vi "PID control.vi"() -> ()   [LabVIEW 2023]
doc: "DESCRIPTION:\n\nThis VI configures the power supply to generate a DC voltage output.\nIt also displays the Output Voltage,Current and Power as per the selected parameter. \n\nINSTRUCTIONS:\n1. Enter the resource name.\n2. Select the desired Channel.\n3. Enter voltage or current value to set the voltage or current value of the power supply .\n4. Set On/Off switch to Enable if you want the generated voltage to appear at the instrument's output. \n5. Select Local/Remote mode operation.If local command is select ,this will set the instrument in local mode.\n6.Select the parameter from the control,to read the responce from the instrument.\n7.Run the VI.\n\nNOTES:\nNotice the order of the power supply component VIs in the block diagram. The first VI in a sequence is the power supply Initialize.vi, which provides a VISA session to the instrument driver. The last VI in a sequence must be the power supply Close.vi which closes the Visa session."
uses:
  <vilib>/Utility/error.llb/DialogType.ctl
  <vilib>/DAQmx/write.llb/DAQmx Write (Digital Bool 1Line 1Point).vi
  <vilib>/DAQmx/read.llb/DAQmx Read (Analog DBL 1Chan 1Samp).vi
  <vilib>/DAQmx/create/channels.llb/DAQmx Create Channel (DO-Digital Output).vi
  <vilib>/DAQmx/miscellaneous.llb/DAQmx Fill In Error Info.vi
  <vilib>/DAQmx/create/channels.llb/DAQmx Create Channel (AI-Voltage-Basic).vi
  <vilib>/addons/control/pid/pid.llb/PID Advanced (DBL).vi
  Downloads/KeithleyKE22xxSeriesVer1.2 (1)/Keithley KE22xx Series/Keithley KE22xx Series.lvlib
  <vilib>/addons/control/pid/NI_PID_pid.lvlib
panel:
  out "message":string=" INSTRUCTIONS:\r\rNormal Use:  When using subVIs that incorporate the error in/error out (or error I/O) structure, place this handler where you want to inform the user of an error, typically at the end of the I/O data path, as the last action of the program.  If the error in error? is ERROR, the handler creates a message describing the error and its source.  If the type of dialog = 1 (default), the message is displayed to the user, who can only acknowedge it.  If the type = 2, the user can acknowledge the message or abort execution; aborting a program with active I/O is not recommended.  If the type = 0, no message is displayed; this is used to process the error programmatically, and the error out cluster elements are wired to individual terminals for that reason.  \r\rOther Use:\n\r\nlocal testing.  To test the error code of a subVI or function that does not have the error I/O structure, you can wire its error code and a source string to the local error code and error source inputs.  If error in error? indicates no error and error code is not equal to 0, the local code and source are substituted for the error in values, and error? is set TRUE (ERROR)."
  in  "stop 2":bool
  out "Temperature [Celsius]\n]":dbl
  in  "Set point Temp [Celsius].":dbl(slide) scale=0.0..40.0
  in  "PID gains in":T1={"proportional gain (Kc)"=1.0, "integral time (Ti, min)"=0.01, "derivative time (Td, min)"=0.0} {"derivative time (Td, min)" format="%.3f"; "integral time (Ti, min)" format="%.3f"; "proportional gain (Kc)" format="%.3f"}
  out "Waveform Chart":T2(graph)
  in  "Channel Select":enum16{"Channel 1", "Channel 2", "Channel 3"}(ring)
  in  "Measurement Function(0:Voltage)":u16(ring) items=["Voltage", "Current", "Power"]
  in  "Function(0:Voltage)":u16(ring) items=["Voltage", "Current"]
  in  "Control Mode(1:Remote)":u16(ring)=1 items=["Local", "Remote"]
  in  "Enable Output (T: Enable)":bool=TRUE
  in  "Unit(V)":u16(ring) items=["V", "mV", "kV", "A", "mA"]
  out "Measurement":string
  in  "VISA resource name":refnum<visa-resource-name>
  # "© 2012 Keithley Instruments, Inc. ALL RIGHTS RESERVED"
  # "Configure Instrument"
  # "Read Measurement"
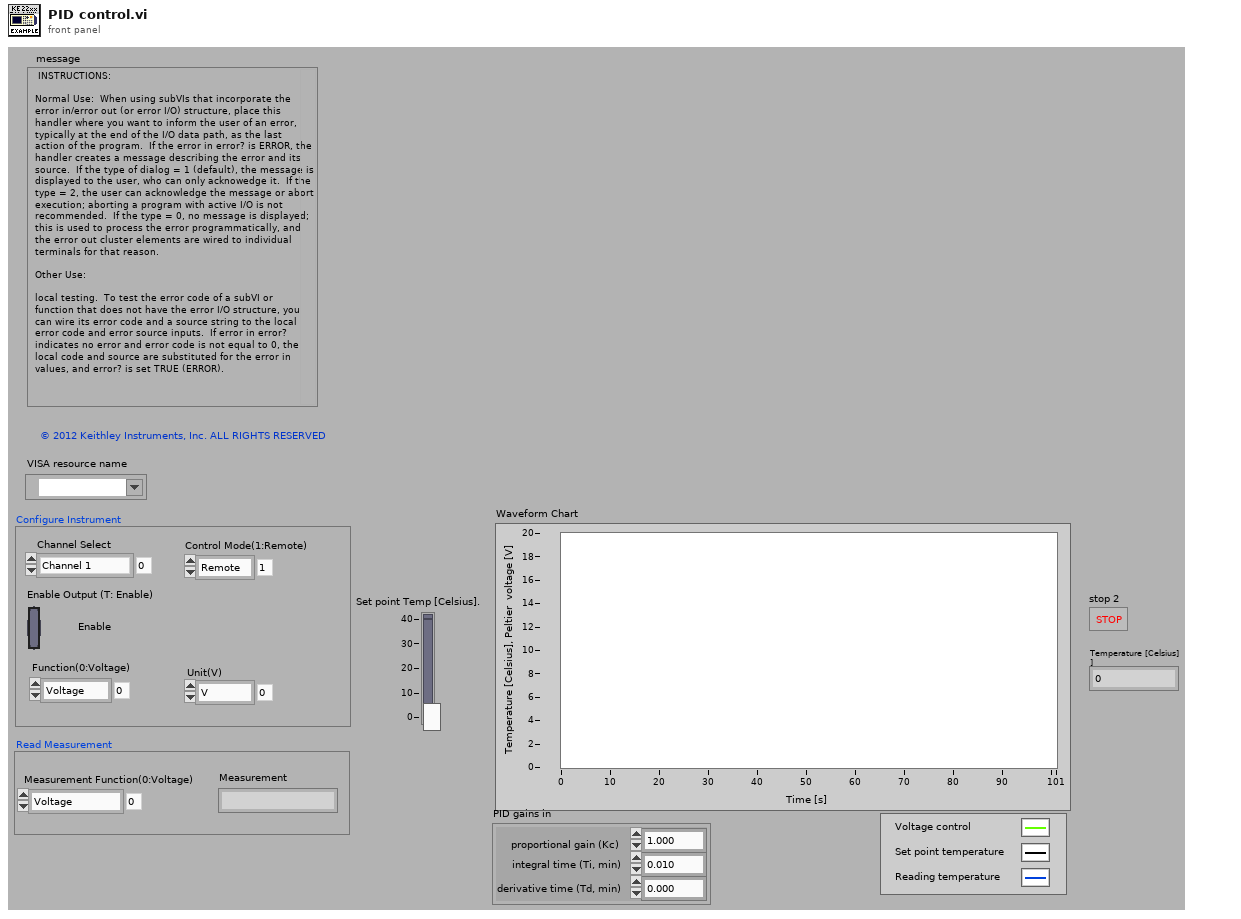
[diagram p1: front panel]
types:
  T1 = cluster{"proportional gain (Kc)":dbl, "integral time (Ti, min)":dbl, "derivative time (Td, min)":dbl}
  T2 = cluster{"Fan Speed":dbl, "Set point Temperature":dbl, "Plant Output":dbl}
  T3 = typedef "DialogType.ctl" = u16
  T4 = cluster{"output":dbl, "Set point Temp [Celsius].":dbl, dbl}
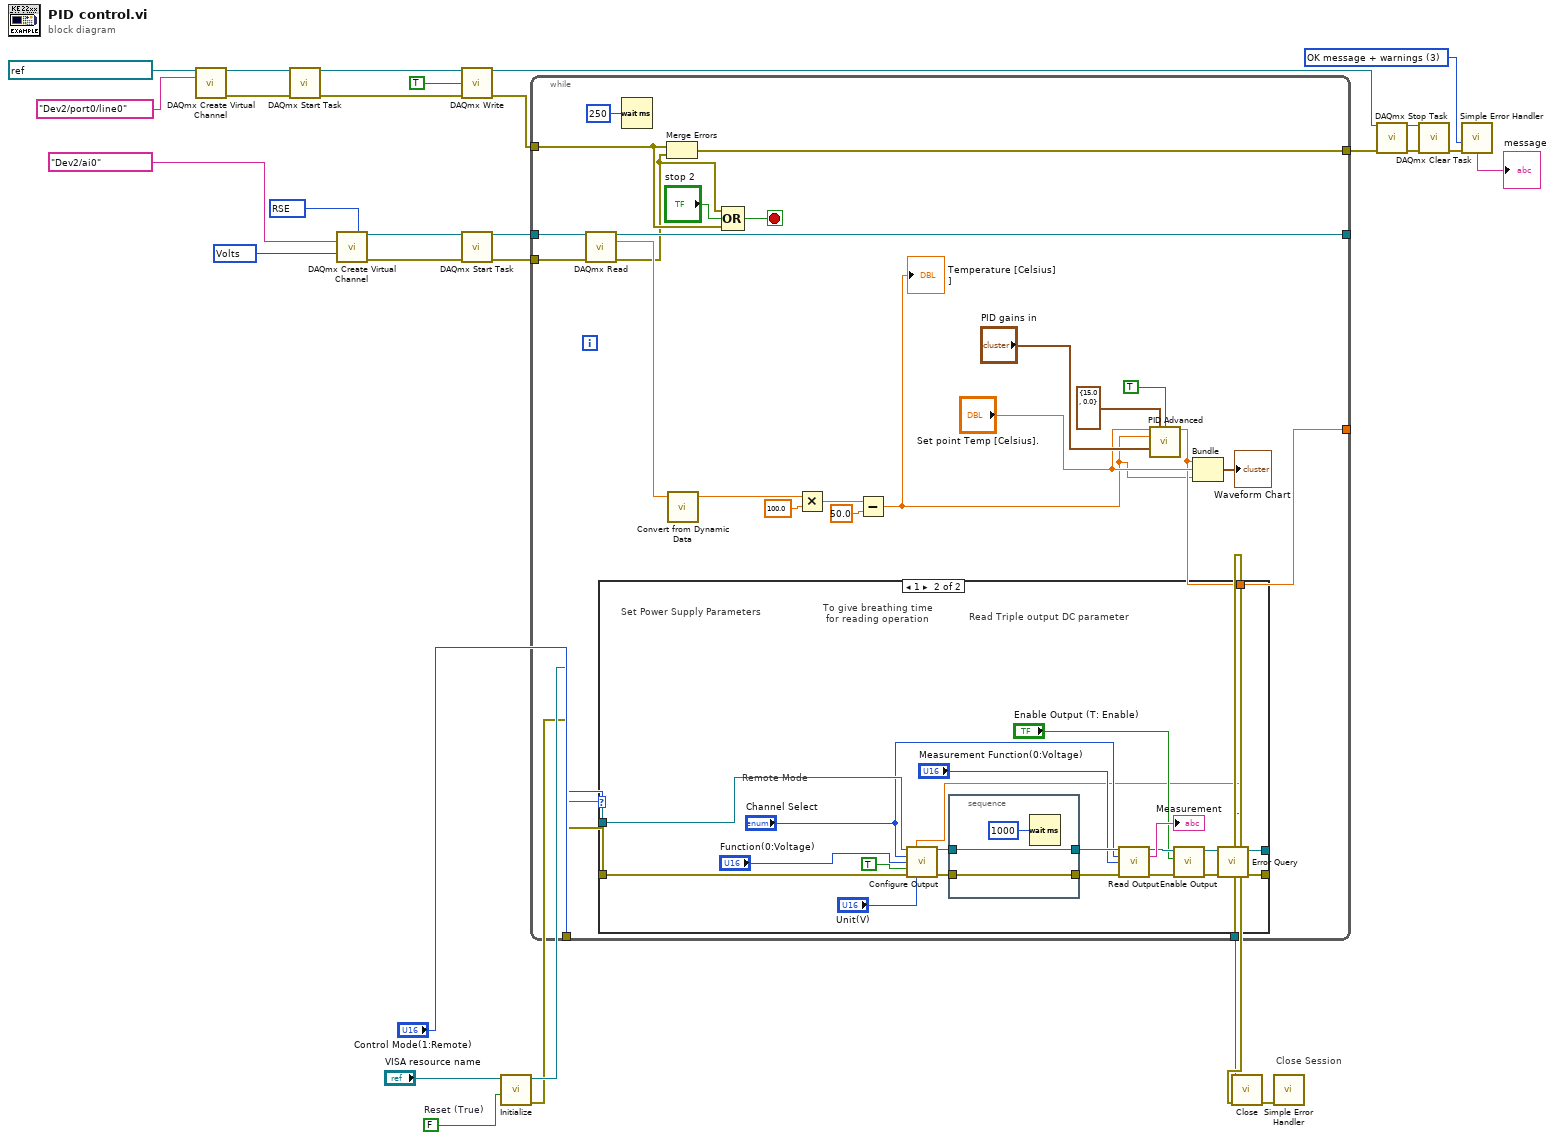
[diagram p0: block diagram]
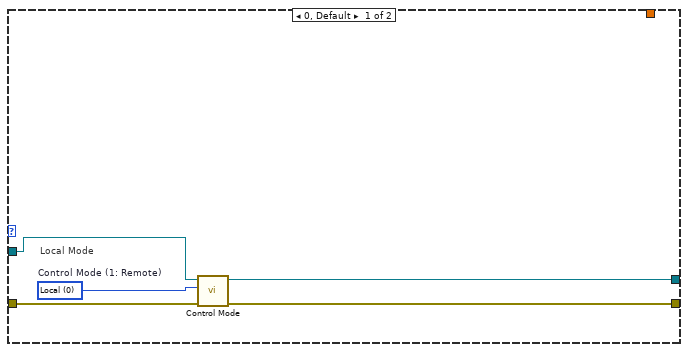
[diagram p2: hidden frame]
diagram:
  w6 = 10083 items=["Default"=-1, "RSE"=10083, "NRSE"=10078, "Differential"=10106, "Pseudodifferential"=12529] ("input terminal configuration")
  w7 = 10348 items=["Volts"=10348, "From Custom Scale"=10065] ("units")
  w11 = T3 3 items=["no dialog", "OK message", "continue or stop message", "OK message + warnings", "continue/stop + warnings"] ("type of dialog (OK msg:1)")
  w28 = FALSE items=["OFF", "ON", "OFF", "ON"]  # Reset (True)
  # "Close Session"
  n1 = call-poly <vilib>:"DAQmx Create Virtual Channel.vi"("task in"=refnum<k21> refnum, "lines"=tag "Dev2/port0/line0") -> ("task out"=w27:refnum<k21>, "error out"=w26:errorcluster)  [unwired: 12 in]
  n2 = call <vilib>:"DAQmx Start Task.vi"("task/channels in"=w27, "error in"=w26) -> ("task out"=w23:refnum<k21>, "error out"=w22:errorcluster)  [unwired: 12 in]
  n3 = call-poly <vilib>:"DAQmx Create Virtual Channel.vi"("input terminal configuration"=w6, "physical channels"=tag "Dev2/ai0", "units"=w7) -> ("task out"=w20:refnum<k21>, "error out"=w19:errorcluster)  [unwired: 11 in]
  n4 = call-poly <vilib>:"DAQmx Write.vi"("task/channels in"=w23, "data"=TRUE, "error in"=w22) -> ("task out"=w10:refnum<k21>, "error out"=w16:errorcluster)  [unwired: 10 in, 1 out]
  n5 = call <vilib>:"DAQmx Start Task.vi"("task/channels in"=w20, "error in"=w19) -> ("task out"=w18:refnum<k21>, "error out"=w17:errorcluster)  [unwired: 12 in]
  n6 = call "Initialize.vi"("Reset (True)"=w28, "VISA resource name"="VISA resource name") -> ("error out"=w3:errorcluster, "VISA resource name out"=w4:refnum<visa-resource-name>)  [unwired: 8 in]
  n7 = while {
    tunnel: w18 -> [w55]
    tunnel: w17 -> [w54]
    tunnel: [w53] -> _
    tunnel: w16 -> [w45]
    tunnel: [w43] -> w9
    tunnel: [w37] -> _
    tunnel: "Control Mode(1:Remote)" -> [w36]
    tunnel: w4 -> [w35]
    tunnel: w3 -> [w34]
    tunnel: [w33] -> w2
    tunnel: [w32] -> w1
    stop <- w48 stop-if-true
    n8 = call-poly <vilib>:"DAQmx Read.vi"("task/channels in"=w55, "error in"=w54) -> ("task out"=w53:refnum<k21>, "data"=w47:dbl, "error out"=w44:errorcluster)  [unwired: 11 in]
    n9 = Wait (ms)(milliseconds to wait=u32 250) -> ()  [unwired: 1 out]
    n10 = Merge Errors(w45, w44) -> (w43:errorcluster)
    n11 = call "Convert from Dynamic Data"("Dynamic Data Type"=w47) -> ("Scalar"=w46:dbl)  [unwired: 3 in]
    n12 = Compound Arithmetic op=OR(w44, "stop 2", w45) -> (w48:bool)
    n13 = Multiply(x=w46, y=100.0) -> (x*y=w51:dbl)
    n14 = Subtract(x=w51, y=50.0) -> (x-y=w31:dbl)
    "Temperature [Celsius]\n]" <- w31
    n15 = call-poly <vilib>:"PID Advanced.vi"("setpoint"="Set point Temp [Celsius].", "output range"=cluster{"output high":dbl, "output low":dbl} {"output high"=15.0, "output low"=0.0}, "auto? (T)"=TRUE, "process variable"=w31, "PID gains"="PID gains in") -> ("output"=w37:dbl)  [unwired: 9 in, 1 out]
    n16 = case shown="1" w36 {
      tunnel: [w58 w72] -> w33
      tunnel: w35 -> [w61 w77]
      tunnel: w34 -> [w60 w76]
      tunnel: [w57 w73] -> w32
      tunnel: w37 -> [_ w62]
      frame 0, Default {
        w59 = u16 0 items=["Local", "Remote", "Remote Lock"]  # Control Mode (1: Remote)
        # "Local Mode"
        n17 = call "Control Mode.vi"("error in (no error)"=w60, "Control Mode (1: Remote)"=w59, "VISA resource name"=w61) -> ("error out"=w58:errorcluster, "VISA resource name out"=w57:refnum<visa-resource-name>)  [unwired: 7 in]
      }
      frame 1 {
        # "Read Triple output DC parameter"
        # "To give breathing time\n for reading operation"
        # "Set Power Supply Parameters"
        # "Remote Mode"
        n18 = call "Configure Output.vi"("VISA resource name"=w77, "Manual Range(0.00)"=w62, "Channel Select"="Channel Select", "Function(0:Voltage)"="Function(0:Voltage)", "Enable Output (T: Enable)"=TRUE, "error in (no error)"=w76, "Unit(V)"="Unit(V)") -> ("VISA resource name out"=w81:refnum<visa-resource-name>, "error out"=w79:errorcluster)  [unwired: 7 in]
        n19 = stacked-sequence {
          tunnel: w81 -> [w83]
          tunnel: [w83] -> w80
          tunnel: w79 -> [w82]
          tunnel: [w82] -> w78
          frame #0 {
            n20 = Wait (ms)(milliseconds to wait=u32 1000 ("millisecond multiple")) -> ()  [unwired: 1 out]
          }
        }
        n21 = call "Read Output.vi"("VISA resource name"=w80, "Channel Select"="Channel Select", "Measurement Function (0:Voltage)"="Measurement Function(0:Voltage)", "error in (no error)"=w78) -> ("VISA resource name out"=w67:refnum<visa-resource-name>, "Measurement"=→"Measurement":string, "error out"=w65:errorcluster)  [unwired: 9 in]
        n22 = call "Enable Output.vi"("error in (no error)"=w65, "Enable Output (T: Enable)"="Enable Output (T: Enable)", "VISA resource name"=w67) -> ("error out"=w64:errorcluster, "VISA resource name out"=w66:refnum<visa-resource-name>)  [unwired: 7 in]
        n23 = call "Error Query.vi"("error in (no error)"=w64, "VISA resource name"=w66) -> ("error out"=w72:errorcluster, "VISA resource name out"=w73:refnum<visa-resource-name>)  [unwired: 6 in, 2 out]
      }
    }
    n24 = Bundle("output"=w37, "Set point Temp [Celsius]."="Set point Temp [Celsius].", w31) -> (→"Waveform Chart":T4)  [unwired: 1 in]
  }
  n25 = call "Close.vi"("error in (no error)"=w2, "VISA resource name"=w1) -> ("error out"=w29:errorcluster)  [unwired: 9 in]
  n26 = call <vilib>:"Simple Error Handler.vi"("error in (no error)"=w29) -> ()  [unwired: 1 in, 8 out]
  n27 = call <vilib>:"DAQmx Stop Task.vi"("task/channels in"=w10, "error in"=w9) -> ("task out"=w15:refnum<k21>, "error out"=w14:errorcluster)  [unwired: 12 in]
  n28 = call <vilib>:"DAQmx Clear Task.vi"("task in"=w15, "error in"=w14) -> ("error out"=w13:errorcluster)  [unwired: 13 in]
  n29 = call <vilib>:"Simple Error Handler.vi"("type of dialog (OK msg:1)"=w11, "error in (no error)"=w13) -> ("message"=→"message":string)  [unwired: 3 in, 4 out]
